vi "Q 2.vi"() -> ()   [LabVIEW 2018]
uses:
  <vilib>/Analysis/5stat.llb/RMS (DBL).vi
  <vilib>/Analysis/baseanly.llb/Mean (DBL).vi
  <vilib>/Analysis/NI_AALBase.lvlib
  <vilib>/Analysis/NI_AALPro.lvlib
panel:
  out "rms value":dbl format="%0.2f"
  out "mean 2":dbl format="%0.2f"
  out "standard deviation":dbl format="%0.2f"
  out "mean":dbl format="%0.2f"
  in  "our index":i32
  in  "Null Array":dbl[](array[numeric])
  out "number (0 to 1)":dbl
  out "Array":dbl[](array[numeric])
  out "Boolean 2":bool
  # "Home work \nQuestion 2\nRandom Number"
  # "Random number"
  # "standard deviation"
  # "show the random number"
  # "will be on if the number be in the range"
  # "Mean"
  # "RMS"
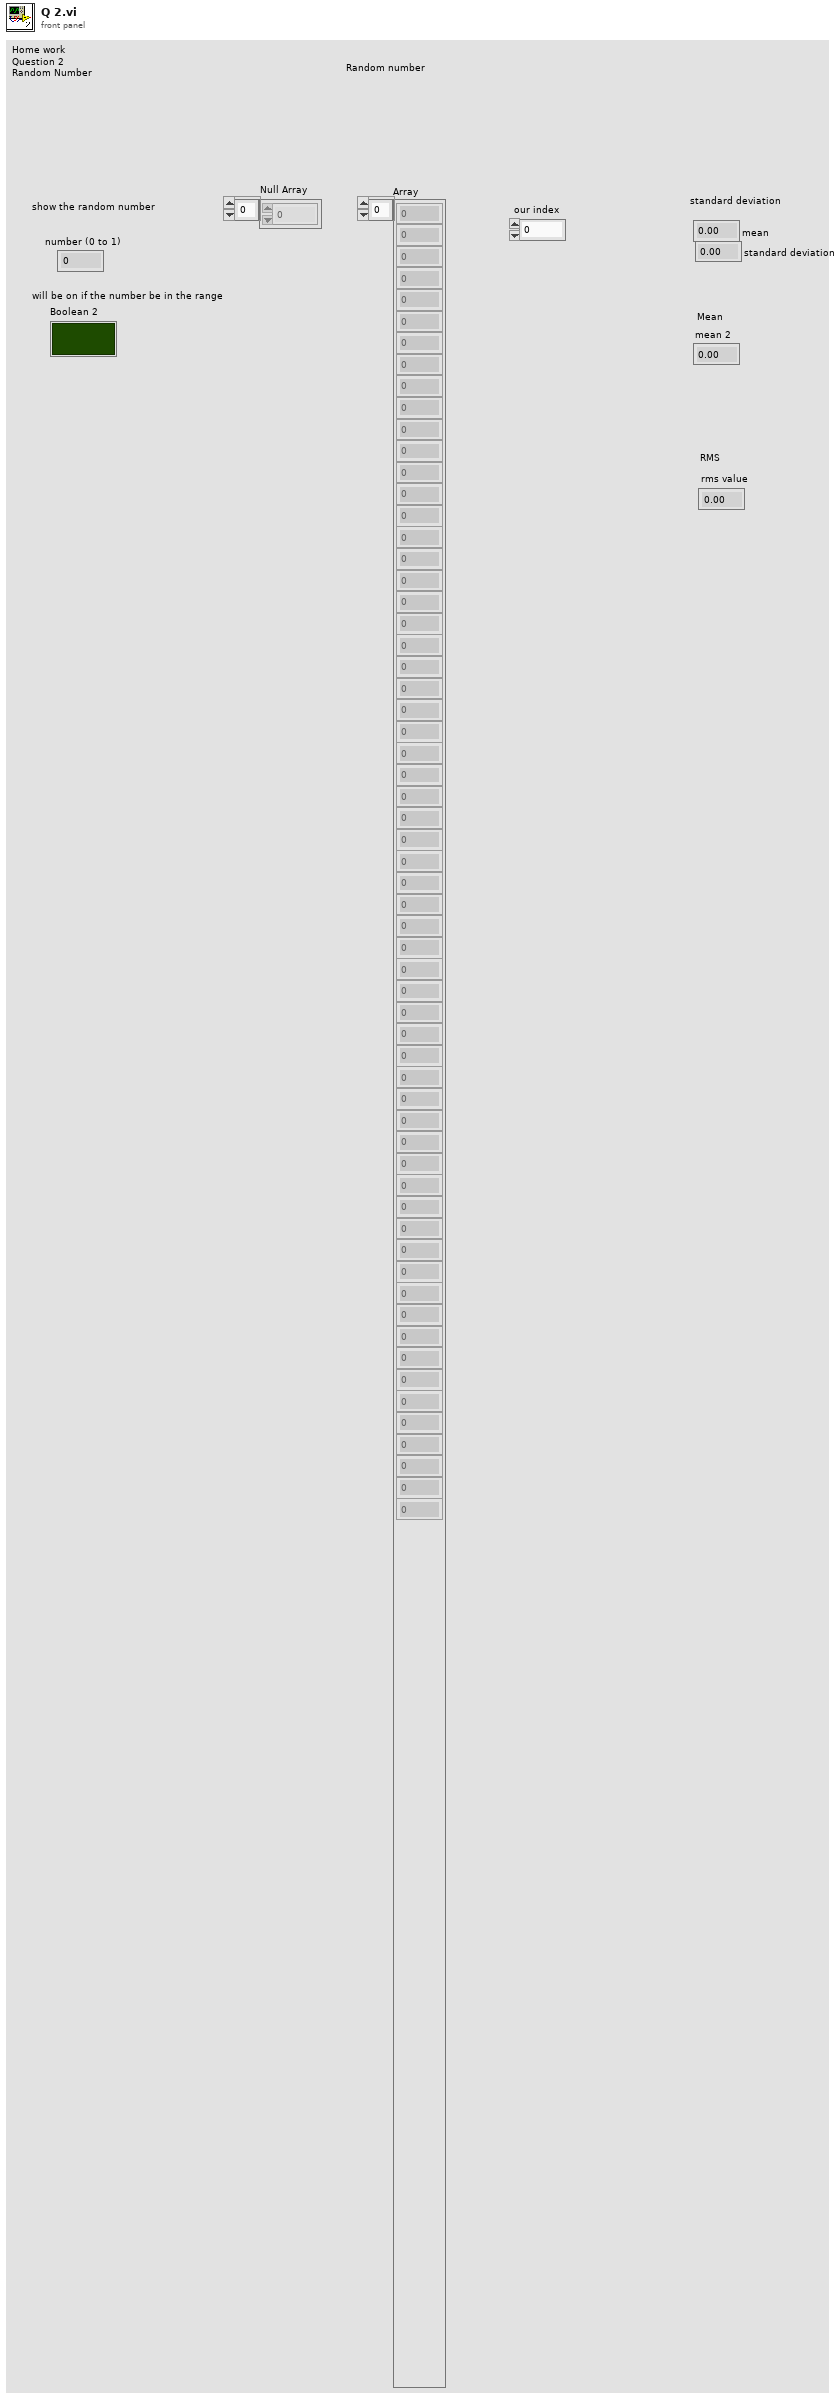
[diagram p1: front panel]
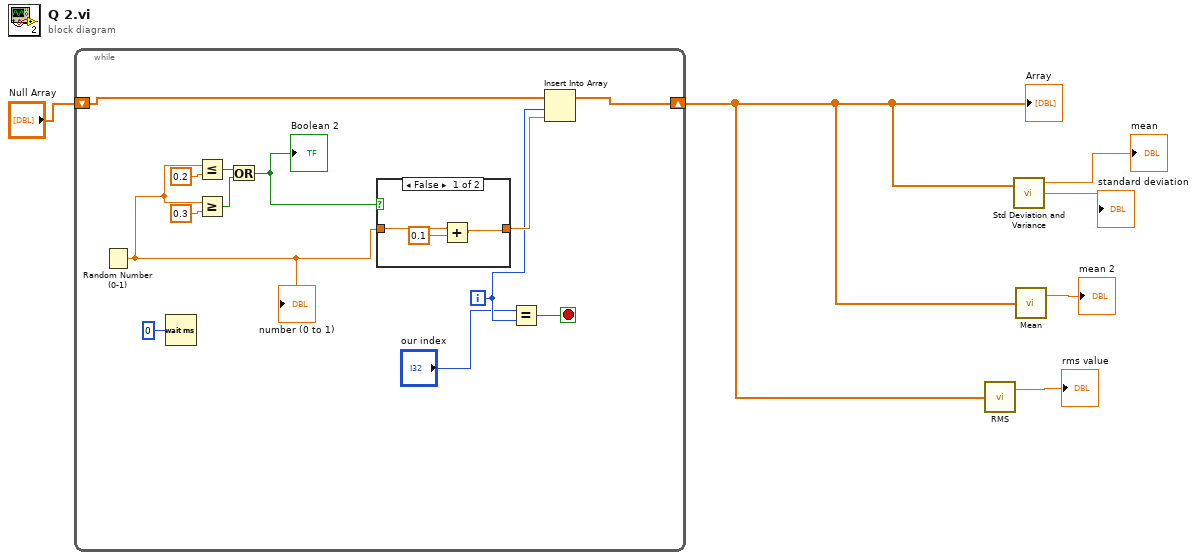
[diagram p0: block diagram]
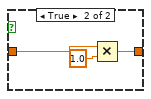
[diagram p2: hidden frame]
diagram:
  n1 = while {
    shift-right: [w10] -> w5
    shift-left: "Null Array" -> [w9]
    i -> [w11]
    stop <- w12 stop-if-true
    n2 = Random Number (0-1)() -> (number: 0 to 1=w8:dbl)
    "number (0 to 1)" <- w8
    n3 = Wait (ms)(milliseconds to wait=u32 0) -> ()  [unwired: 1 out]
    n4 = Less Or Equal?(x=w8, y=0.2) -> (x <= y?=w16:bool)
    n5 = Greater Or Equal?(x=w8, y=0.3 ("output variable")) -> (x >= y?=w15:bool)
    n6 = Or(x=w16, y=w15) -> (x .or. y?=w14:bool)
    "Boolean 2" <- w14
    n7 = case shown="False" w14 {
      tunnel: w8 -> [w20 w24]
      tunnel: [w21 w25] -> w13
      frame False {
        n8 = Add(x=w20, y=0.1) -> (x+y=w21:dbl)
      }
      frame True {
        n9 = Multiply(x=w24, y=1.0) -> (x*y=w25:dbl)
      }
    }
    n10 = Equal?(x="our index", y=w11) -> (x = y?=w12:bool)
    n11 = Insert Into Array(array=w9, index=w11, new element=w13) -> (w10:dbl[])
  }
  "Array" <- w5
  n12 = call-poly <vilib>:"RMS.vi"("X"=w5) -> ("rms value"=→"rms value":dbl)  [unwired: 1 out]
  n13 = call <vilib>:"Std Deviation and Variance.vi"("X"=w5) -> ("mean"=→"mean":dbl, "standard deviation"=→"standard deviation":dbl)  [unwired: 1 in, 1 out]
  n14 = call-poly <vilib>:"Mean.vi"("X"=w5) -> ("mean"=→"mean 2":dbl)  [unwired: 1 out]
